vi "VoltageTest_L_VDC20V-2.vi"(0 "datain":string[](array[string])=["备注", "负载通道", "负载地址", "延时时间", "output max", "output min", "量测类型", "待测物板号"], 5 "HW CH Number":i32, 7 "Setup":string) -> (4 "REPORT INDECATE":string[][](array[string])=[["微安测试", "", "", "", ""], ["微安量测", "4", "0.000", "0.1", "NG"], ["微安量测", "4", "0.000", "0.1", "NG"], ["微安量测", "4", "0.000", "0.1", "NG"], ["微安量测", "4", "0.000", "0.1", "NG"]], 6 "ROW HEAD":string[](array[string]), 8 "PF":string[](array[string]), 10 "testData":string[](array[string]), 15 "Array":string[](array[string]))   [LabVIEW 2018]
uses:
  Subvi/Global.vi
panel:
  in  "error in (no error)":errorcluster caption="错误输入（无错误）"
  out "error out":errorcluster
  out "测试板数":i32
  out "数组":bool[](array[boolean])
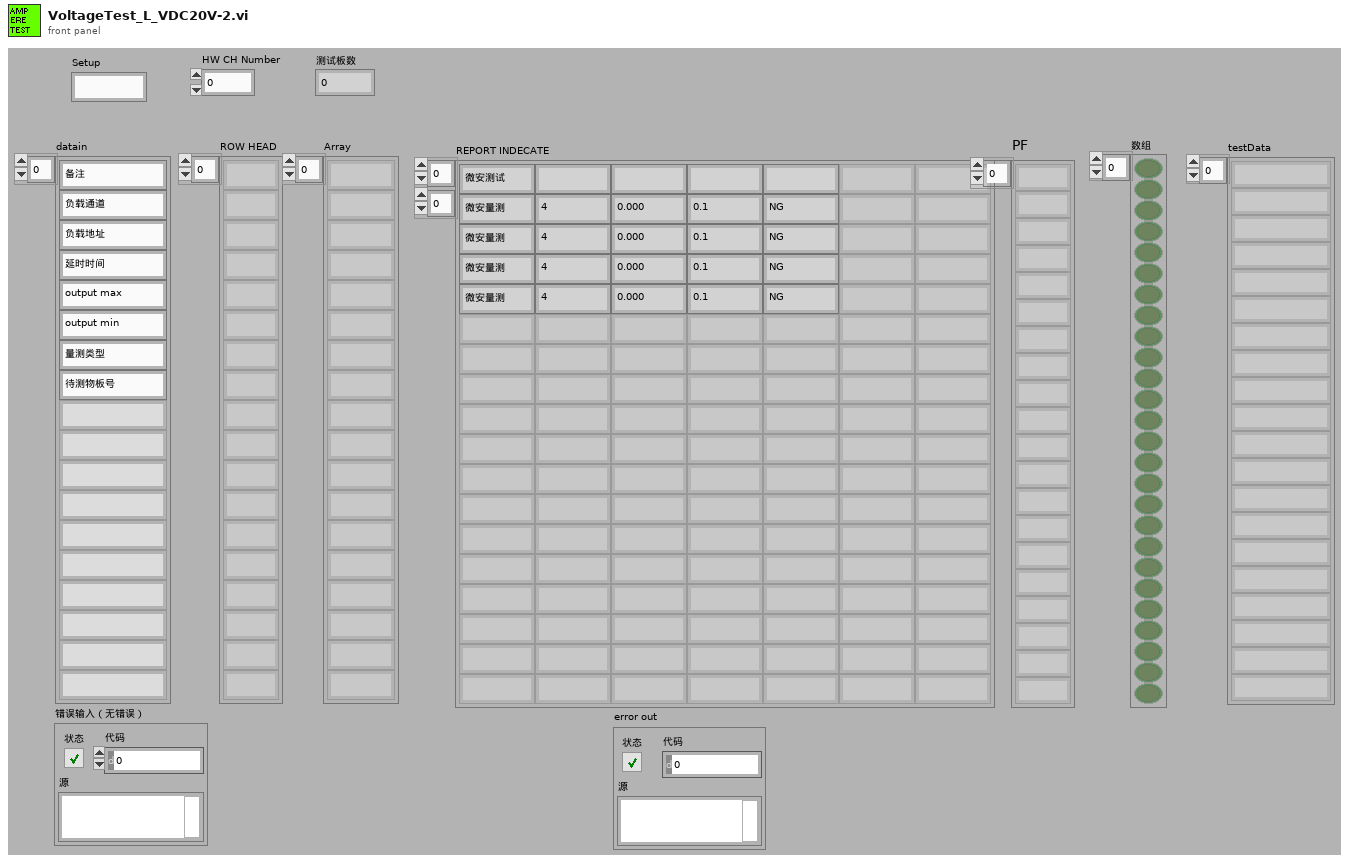
[diagram p1: front panel]
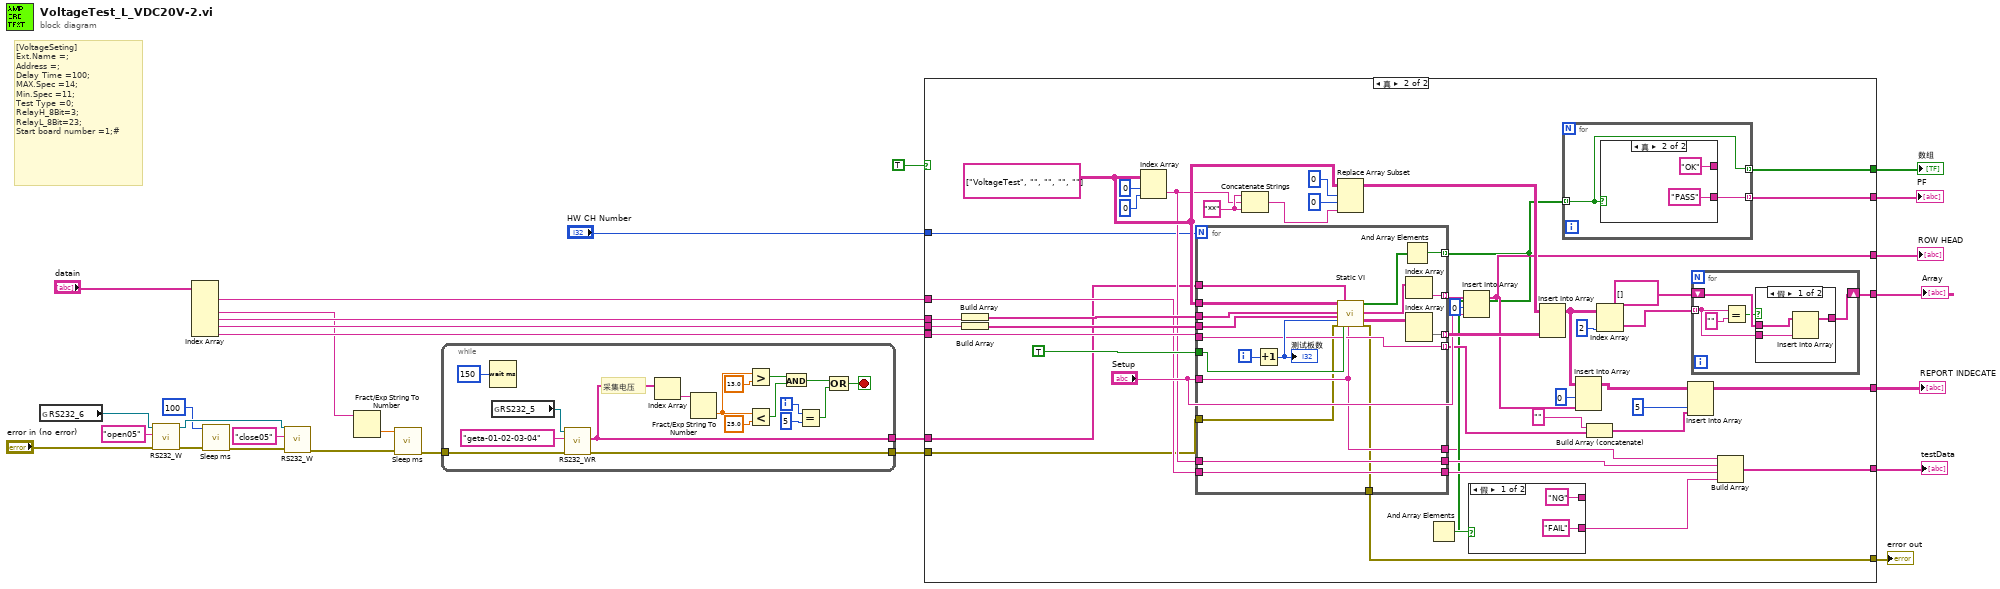
[diagram p0: block diagram]
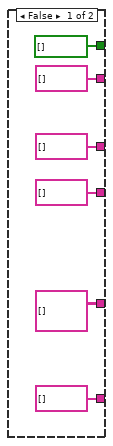
[diagram p2: hidden frame]
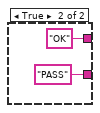
[diagram p3: hidden frame]
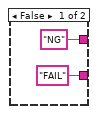
[diagram p4: hidden frame]
diagram:
  # "[VoltageSeting]\nExt.Name =;\nAddress =;\nDelay Time =100;\nMAX.Spec =14;\nMin.Spec =11;\nTest Type =0;\nRelayH_8Bit=3;\nRelayL_8Bit=23;\nStart board number =1;#"
  n1 = global read "Global.vi" "RS232_6"() -> (w14:refnum<visa-resource-name>)
  n2 = call "RS232_W.vi"("error in (no error)"="error in (no error)", "CMD"="open05", "VISA资源名称"=w14) -> ("error out"=w11:errorcluster, "VISA资源名称输出"=w13:refnum<visa-resource-name>)  [unwired: 6 in, 1 out]
  n3 = Index Array(array="datain") -> (element #1=w20:string, element #3=w5:string, element #4=w25:string, element #5=w24:string, element #6=w22:string)  [unwired: 6 in, 1 out]
  n4 = call "Sleep ms.vi"("error in (no error)"=w11, "等待时间（毫秒）"=u32 100) -> ("error out"=w12:errorcluster)  [unwired: 9 in]
  n5 = call "RS232_W.vi"("error in (no error)"=w12, "CMD"="close05", "VISA资源名称"=w13) -> ("error out"=w6:errorcluster)  [unwired: 6 in, 2 out]
  n6 = Fract/Exp String To Number(string=w5) -> (number=w7:dbl)  [unwired: 3 in, 1 out]
  n7 = call "Sleep ms.vi"("error in (no error)"=w6, "等待时间（毫秒）"=w7) -> ("error out"=w4:errorcluster)  [unwired: 9 in]
  n8 = while {
    tunnel: [w32] -> w16
    tunnel: w4 -> [w31]
    tunnel: [w29] -> w3
    i -> [w33]
    stop <- w34 stop-if-true
    # "采集电压"
    n9 = Wait (ms)(milliseconds to wait=u32 150 ("等待时间（毫秒）")) -> ()  [unwired: 1 out]
    n10 = global read "Global.vi" "RS232_5"() -> (w44:refnum<visa-resource-name>)
    n11 = call "RS232_WR.vi"("error in (no error)"=w31, "CMD"="geta-01-02-03-04", "VISA资源名称"=w44) -> ("error out"=w29:errorcluster, "Out data"=w32:string[])  [unwired: 6 in, 1 out]
    n12 = Index Array(array=w32) -> (element=w35:string)  [unwired: 1 in]
    n13 = Fract/Exp String To Number(string=w35) -> (number=w37:dbl)  [unwired: 3 in, 1 out]
    n14 = Greater?(x=w37, y=13.0) -> (0:w39:bool)
    n15 = Less?(x=w37, y=25.0) -> (x < y?=w40:bool)
    n16 = And(x=w39, y=w40) -> (x .and. y?=w38:bool)
    n17 = Equal?(x=w33, y=5) -> (x = y?=w43:bool)
    n18 = Compound Arithmetic op=OR ("复合运算")(w38, w43) -> (w34:bool)
  }
  n19 = case shown="真" TRUE {
    tunnel: [string[] [] ("Array") w94] -> w28
    tunnel: [string[] [] w93] -> w27
    tunnel: w25 -> [_ w86]
    tunnel: w24 -> [_ w85]
    tunnel: [string[] [] w74] -> w23
    tunnel: w22 -> [_ w72]
    tunnel: [string[][] [] w69] -> w21
    tunnel: w20 -> [_ w64]
    tunnel: [string[] [] w58] -> w19
    tunnel: [bool[] [] w56] -> w18
    tunnel: "HW CH Number" -> [_ w55]
    tunnel: w16 -> [_ w54]
    tunnel: w3 -> [_ w53]
    tunnel: [_ w52] -> w2
    frame False {
    }
    frame True {
      w84 = string[][] [["VoltageTest", "", "", "", ""]]
      w90 = "**" ("字符串")
      n20 = Build Array(w86) -> (w83:string[])
      n21 = Build Array(w85) -> (w82:string[])
      n22 = Index Array(array=w84, index (row)=0 ("索引 (行)"), index (col)=0 ("禁用的索引 (列)")) -> (element=w65:string)
      n23 = for {
        N: w55 -> [_]
        tunnel: w54 -> [w120]
        tunnel: w83 -> [w118]
        tunnel: w82 -> [w117]
        tunnel: "Setup" -> [w104]
        tunnel: TRUE -> [w115]
        tunnel: [w113] -> w60 mode=indexing
        tunnel: [w110] -> w78 mode=indexing
        tunnel: w84 -> [w119]
        tunnel: [w108] -> w79 mode=indexing
        tunnel: w72 -> [w107]
        tunnel: [w107] -> w68 mode=indexing
        tunnel: w65 -> [w106]
        tunnel: [w106] -> w63
        tunnel: w64 -> [w105]
        tunnel: [w105] -> w62
        tunnel: [w104] -> w57
        tunnel: w53 -> [w103]
        tunnel: [w102] -> w52
        i -> [w112]
        n24 = Increment(x=w112) -> (x+1=w114:i32)
        "测试板数" <- w114
        n25 = call "Static VI.vi"("添加的数组"=w119, "Max"=w118, "Min"=w117, "板数"=w114, "error in (no error)"=w103, "INPUTSTRING"=w120, "是否为字符串对比"=w115, "SQ"=w104) -> ("P/F"=w116:bool[], "SQ out"=w111:string[], "arrauy out"=w109:string[][], "error out"=w102:errorcluster)  [unwired: 8 in]
        n26 = And Array Elements(Boolean array=w116) -> (logical AND=w113:bool)
        n27 = Index Array(array=w111) -> (element=w110:string)  [unwired: 1 in]
        n28 = Index Array(array=w109) -> (element=w108:string[])  [unwired: 2 in]
      }
      n29 = Concatenate Strings(w90, w65, w90) -> (w87:string)
      n30 = Replace Array Subset(array=w84, new element=w87, index (row)=0 ("索引 (行)"), index (col)=0 ("禁用的索引 (列)")) -> (w80:string[][])
      n31 = And Array Elements(Boolean array=w60) -> (logical AND=w61:bool)
      n32 = Insert Into Array(array=w78, index=0 ("索引"), new element="Setup") -> (w74:string[])
      n33 = case shown="假" w61 {
        tunnel: ["NG" "OK"] -> _
        tunnel: ["FAIL" "PASS"] -> w59
        frame False {
        }
        frame True {
        }
      }
      n34 = Insert Into Array ("数组插入")(array=w80, new element=w79) -> (w75:string[][])  [unwired: 2 in]
      n35 = for {
        tunnel: w60 -> [w121] mode=indexing
        tunnel: [w122] -> w93 mode=indexing
        tunnel: [w121] -> w56 mode=indexing
        n36 = case shown="真" w121 {
          tunnel: ["NG" "OK"] -> _
          tunnel: ["FAIL" "PASS"] -> w122
          frame False {
          }
          frame True {
          }
        }
      }
      n37 = Insert Into Array(array=w75, index (col)=0 ("禁用的索引 (列)"), new element=w74) -> (w70:string[][])  [unwired: 1 in]
      n38 = Build Array (concatenate)("" ("字符串"), w68) -> (w66:string[])
      n39 = Index Array(array=w75, index (col)=2 ("禁用的索引 (列)")) -> (element=w95:string[])  [unwired: 1 in]
      n40 = Insert Into Array(array=w70, index (col)=5 ("禁用的索引 (列)"), new element=w66) -> (w69:string[][])  [unwired: 1 in]
      n41 = for {
        tunnel: w95 -> [w127] mode=indexing
        shift-right: [w128] -> w94
        shift-left: string[] [] ("Array") -> [w131]
        n42 = Equal?(x=w127, y="") -> (x = y?=w129:bool)
        n43 = case shown="假" w129 {
          tunnel: w131 -> [w134 w135]
          tunnel: [w133 w135] -> w128
          tunnel: w127 -> [w132 _]
          frame False {
            n44 = Insert Into Array(array=w134, new element=w132) -> (w133:string[])  [unwired: 1 in]
          }
          frame True {
          }
        }
      }
      n45 = Build Array(w57, w63, w62, w59) -> (w58:string[])
    }
  }
  "REPORT INDECATE" <- w21
  "ROW HEAD" <- w23
  "PF" <- w27
  "Array" <- w28
  "数组" <- w18
  "testData" <- w19
  "error out" <- w2
